vi "ReaderDaemon.vi"(6 "E-Stop DVR":refnum<data-value>, 8 "error in (no error)":errorcluster, 9 "Connected? DVR":refnum<data-value>, 10 "Variant Queue":T1, 11 "Reader Parameters":T2={"reader name"="", "writer url"="", "reader buffer size"=-1}) -> (0 "error out":errorcluster)   [LabVIEW 2013, in "NetworkStreamReader.lvclass"]
doc: "Daemon (running in the background) which consistently checks the reader endpoint to see if a new value is available, and then passes it into the internal queue of the NetworkStreamReader if data is available. If the network stream is disconnected, it will attempt to reconnect until the connection is reestablished or the Close method is called.\n\n<b>This VI must be stopped by calling the Close method of the Object which launched it.</b>\n\nJared Kirschner, 2012."
uses:
  NetworkStreamReader.lvclass
  ReaderParameters.ctl
  Shared/TimeStampedMessageQueue.ctl
  Shared/TimeStampedMessage.ctl
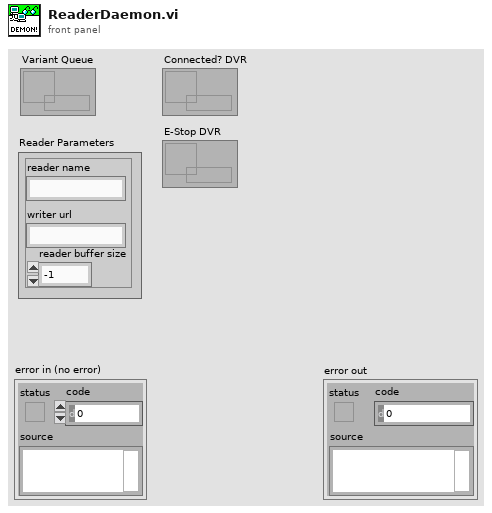
[diagram p1: front panel]
types:
  T1 = typedef "TimeStampedMessageQueue.ctl" = refnum<queue>
  T2 = typedef "NetworkStreamReader.lvclass/ReaderParameters.ctl" = cluster{"reader name":string, "writer url":string, "reader buffer size":i32}
  T3 = typedef "ElapsedTimeMessage.ctl" = cluster{"Data":variant, "Elapsed Time (s)":dbl}
  T4 = typedef "TimeStampedMessage.ctl" = cluster{"Data":variant, "Time Stamp":timestamp}
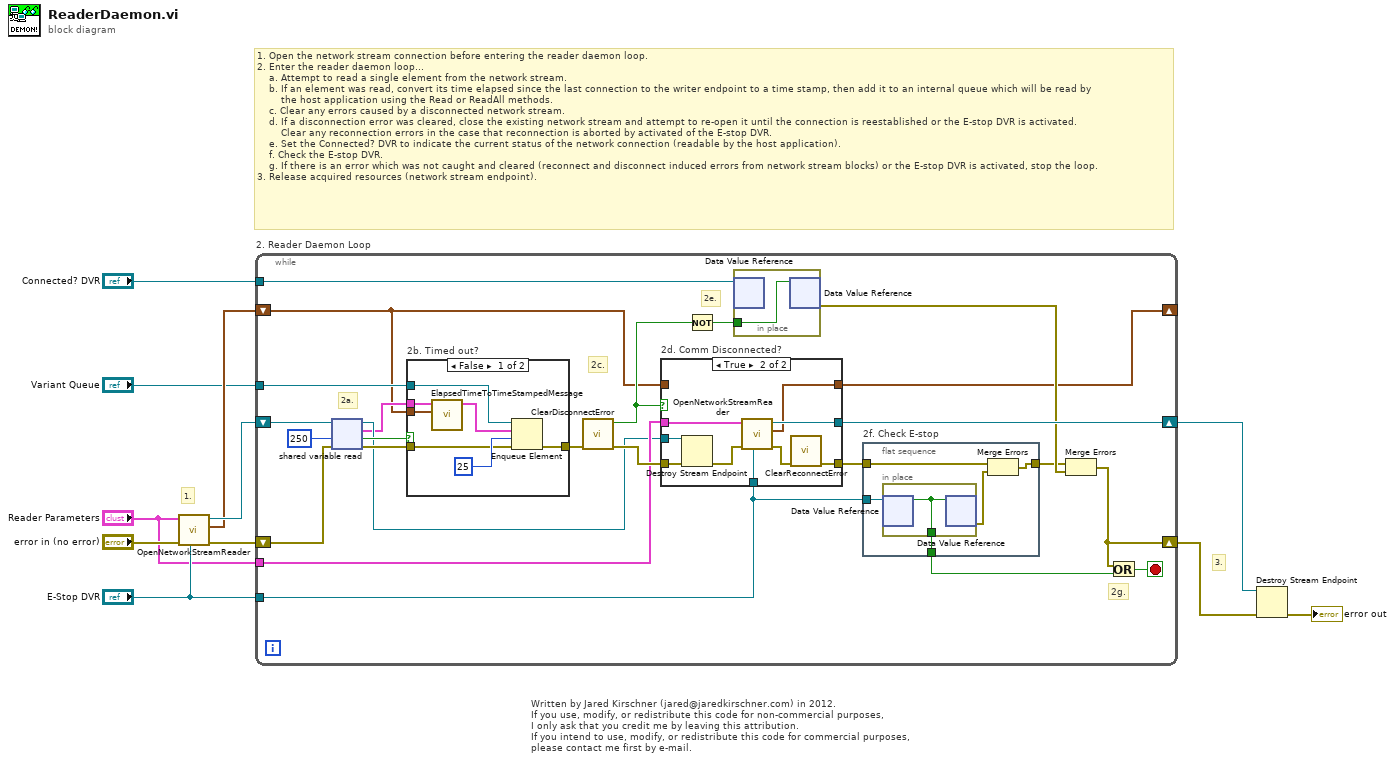
[diagram p0: block diagram]
diagram:
  # "1. Open the network stream connection before entering the reader daemon loop.\n2. Enter the reader daemon loop...\n    a. Attempt to read a single element from the network stream.\n    b. If an element was read, convert its time elapsed since the last connection to the writer endpoint to a time stamp, then add it to an internal queue which will be read by\n        the host application using the Read or ReadAll methods.\n    c. Clear any errors caused by a disconnected network stream.\n    d. If a disconnection error was cleared, close the existing network stream and attempt to re-open it until the connection is reestablished or the E-stop DVR is activated.\n        Clear any reconnection errors in the case that reconnection is aborted by activated of the E-stop DVR.\n    e. Set the Connected? DVR to indicate the current status of the network connection (readable by the host application).\n    f. Check the E-stop DVR.\n    g. If there is an error which was not caught and cleared (reconnect and disconnect induced errors from network stream blocks) or the E-stop DVR is activated, stop the loop.\n3. Release acquired resources (network stream endpoint)."
  # "3."
  # "1."
  # "Written by Jared Kirschner (jared@jaredkirschner.com) in 2012.\nIf you use, modify, or redistribute this code for non-commercial purposes,\nI only ask that you credit me by leaving this attribution.\nIf you intend to use, modify, or redistribute this code for commercial purposes,\nplease contact me first by e-mail."
  n1 = call "OpenNetworkStreamReader.vi"("E-Stop DVR"="E-Stop DVR", "error in (no error)"="error in (no error)", "Reader Parameters"="Reader Parameters") -> ("error out"=w9:errorcluster, "Time Opened"=w2:timestamp, "Reader Endpoint"=w10:refnum<k21>)  [unwired: 5 in, 1 out]
  n2 = while "2. Reader Daemon Loop" {
    tunnel: "Variant Queue" -> [w32]
    shift-right: [w19] -> w3
    shift-left: w9 -> [w29]
    shift-right: [w25] -> w5
    shift-left: w10 -> [w30]
    tunnel: "E-Stop DVR" -> [w21]
    tunnel: "Connected? DVR" -> [w28]
    tunnel: "Reader Parameters" -> [w26]
    shift-right: [w14] -> _
    shift-left: w2 -> [w12]
    stop <- w23 stop-if-true
    # "2g."
    # "2e."
    # "2c."
    # "2a."
    n3 = shared-variable-read(w30, w29, 250 ("timeout in ms (-1)")) -> (w24:refnum<k21>, w34:errorcluster, w33:bool, w13:T3)
    n4 = case "2b. Timed out?" shown="False" w33 {
      tunnel: w34 -> [w59 w62]
      tunnel: w32 -> [w61 _]
      tunnel: [w58 w62] -> w31
      tunnel: w13 -> [w56 _]
      tunnel: w12 -> [w55 _]
      frame False {
        n5 = call "ElapsedTimeToTimeStampedMessage.vi"("Time Opened"=w55, "ElapsedTimeMessage"=w56) -> ("TimeStampedMessage"=w57:T4)  [unwired: 9 in]
        n6 = Enqueue Element(queue=w61, element=w57, timeout in ms (-1)=25, error in (no error)=w59) -> (error out=w58:errorcluster)  [unwired: 2 out]
      }
      frame True {
      }
    }
    n7 = call "ClearDisconnectError.vi"("error in (no error)"=w31) -> ("error out"=w27:errorcluster, "Disconnect error?"=w16:bool)  [unwired: 9 in]
    n8 = case "2d. Comm Disconnected?" shown="True" w16 {
      tunnel: w21 -> [_ w53]
      tunnel: w27 -> [w43 w48]
      tunnel: w26 -> [_ w52]
      tunnel: [w44 w51] -> w25
      tunnel: w24 -> [w44 w50]
      tunnel: [w43 w46] -> w22
      tunnel: w12 -> [w42 _]
      tunnel: [w42 w45] -> w14
      frame False {
      }
      frame True {
        n9 = Destroy Stream Endpoint(8:w48, 11:w50) -> (0:w49:errorcluster)
        n10 = call "OpenNetworkStreamReader.vi"("E-Stop DVR"=w53, "error in (no error)"=w49, "Reader Parameters"=w52) -> ("error out"=w47:errorcluster, "Time Opened"=w45:timestamp, "Reader Endpoint"=w51:refnum<k21>)  [unwired: 5 in, 1 out]
        n11 = call "ClearReconnectError.vi"("error in (no error)"=w47) -> ("error out"=w46:errorcluster)  [unwired: 9 in, 1 out]
      }
    }
    n12 = Not(x=w16) -> (.not. x?=w15:bool)
    n13 = in-place {
      in-place-border: w15 -> [w54]
      n14 = in-place-dvr #1(w28) -> ()  [unwired: 2 out]
      n15 = in-place-dvr #1(w54) -> (w18:errorcluster)  [unwired: 1 out]
    }
    n16 = flat-sequence "2f. Check E-stop" {
      tunnel: w22 -> [w37]
      tunnel: w21 -> [w40]
      tunnel: [w39] -> w20
      tunnel: [w38] -> w17
      frame #0 {
        n17 = in-place {
          in-place-border: [w41] -> w39
          n18 = in-place-dvr #2(w40) -> (w41:bool)  [unwired: 1 out]
          n19 = in-place-dvr #2(w41) -> (w36:errorcluster)  [unwired: 1 out]
        }
        n20 = Merge Errors(w37, w36) -> (w38:errorcluster)
      }
    }
    n21 = Merge Errors(w17, w18) -> (w19:errorcluster)
    n22 = Or(x=w19, y=w20) -> (x .or. y?=w23:bool)
  }
  n23 = Destroy Stream Endpoint(8:w3, 11:w5) -> (0:→"error out":errorcluster)
